vi "ringbuffer.vi"(8 "new val":dbl, 9 "index in":i32, 10 "array size":i32, 11 "array in":dbl[](array[numeric])) -> (1 "index out":i32, 3 "array out":dbl[](array[numeric]))   [LabVIEW 2017]
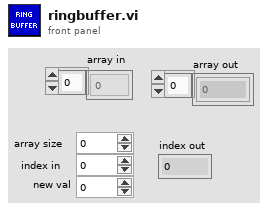
[diagram p1: front panel]
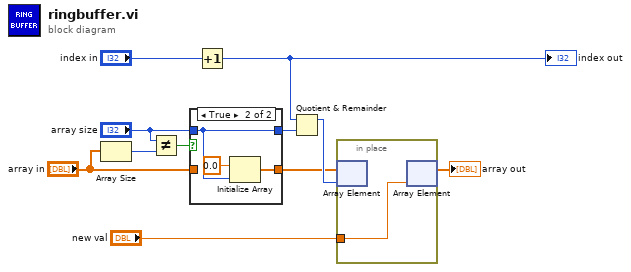
[diagram p0: block diagram]
diagram:
  n1 = Array Size(array="array in") -> (size(s)=w6:i32)
  n2 = Not Equal?(x="array size", y=w6) -> (x != y?=w9:bool)
  n3 = case shown="True" w9 {
    tunnel: [w13 w15] -> w8
    tunnel: "array in" -> [w13 _]
    tunnel: "array size" -> [w12 w14]
    tunnel: [w12 w14] -> w4
    frame False {
    }
    frame True {
      n4 = Initialize Array(0.0 ("element"), w14) -> (w15:dbl[])
    }
  }
  n5 = Increment(x="index in") -> (x+1=w1:i32)
  "index out" <- w1
  n6 = Quotient & Remainder(x=w1, y=w4) -> (x-y*floor(x/y)=w11:i32)  [unwired: 1 out]
  n7 = in-place {
    in-place-border: "new val" -> [w17]
    n8 = in-place-array #1(w8, w11) -> ()  [unwired: 1 out]
    n9 = in-place-array #1(w17) -> (→"array out":dbl[])  [unwired: 1 out]
  }
